vi "MasterSample Info_DL.vi"(8 "error in (no error)":errorcluster, 10 "MasterSampleInfo":T1, 11 "DataLogger in":refnum<class "DataLogger.lvclass">) -> (0 "error out":errorcluster, 3 "DataLogger out":refnum<class "DataLogger.lvclass">)   [LabVIEW 2019, in "DataLogger.lvclass"]
uses:
  DataLogger.lvclass
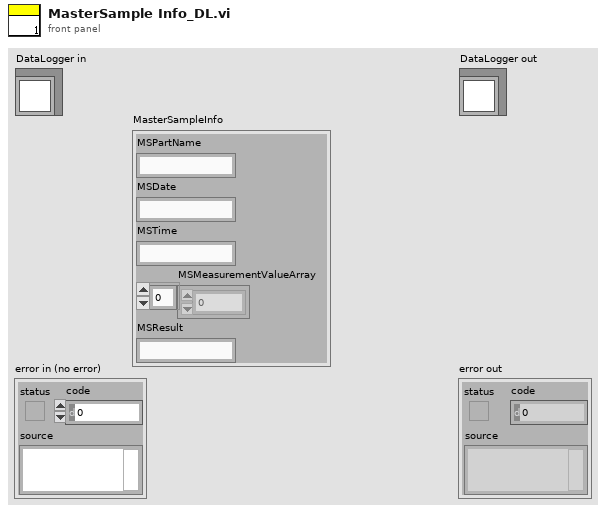
[diagram p1: front panel]
types:
  T1 = cluster{"MSPartName":string, "MSDate":string, "MSTime":string, "MSMeasurementValueArray":dbl[], "MSResult":string}
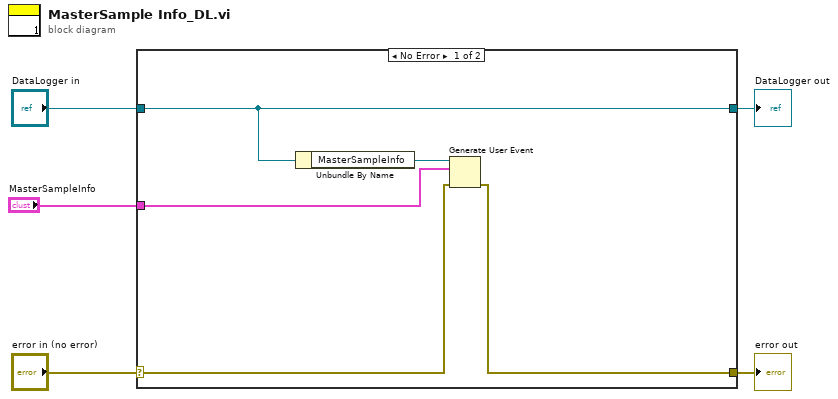
[diagram p0: block diagram]
diagram:
  n1 = case shown="No Error" "error in (no error)" {
    selector: "error in (no error)" -> [w8 w12]
    tunnel: [w7 w12] -> w4
    tunnel: [w10 w11] -> w2
    tunnel: "DataLogger in" -> [w10 w11]
    tunnel: "MasterSampleInfo" -> [w6 _]
    frame No Error {
      n2 = Unbundle By Name(w10) -> ("MasterSampleInfo"=w9:refnum<user-event>)
      n3 = Generate User Event(user event=w9, event data cluster=w6, error in=w8) -> (error out=w7:errorcluster)  [unwired: 1 in, 1 out]
    }
    frame Error {
    }
  }
  "error out" <- w4
  "DataLogger out" <- w2
